vi "Send Command.vi"(8 "error in (no error)":errorcluster, 10 "Consumer Queues in":T1, 11 "Trig Process Command":refnum<class "Generic Trig Process Command.lvclass">) -> (0 "error out":errorcluster, 2 "Consumer Queues out":T1)   [LabVIEW 2019, in "Trig Process.lvlib" / "Generic Trig Process Command.lvclass"]
uses:
  Generic Trig Process Command.lvclass
  TS Framework/Consumer Queues.ctl
  UI Process/Generic UI Command/Generic UI Process Command.lvclass
  DAC Process/Generic DAC Command/Generic DAC Process Command.lvclass
  TS Framework/TS Framework.lvlib
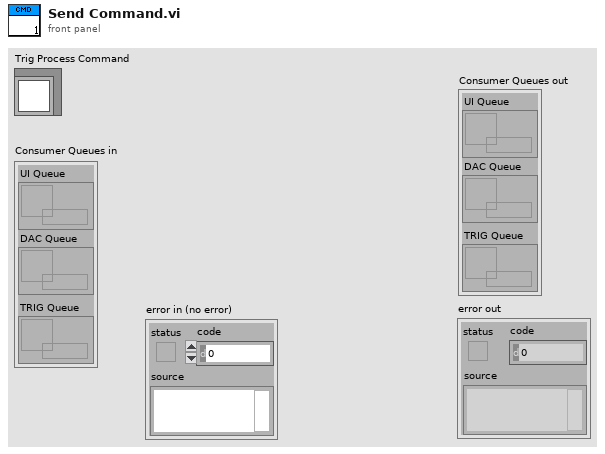
[diagram p1: front panel]
types:
  T1 = typedef "TS Framework.lvlib/Consumer Queues.ctl" = cluster{"UI Queue":refnum<queue>, "DAC Queue":refnum<queue>, "TRIG Queue":refnum<queue>}
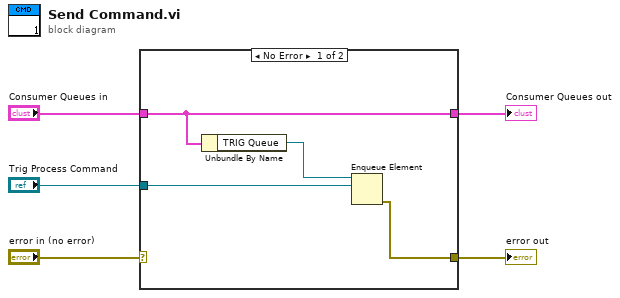
[diagram p0: block diagram]
diagram:
  n1 = case shown="No Error" "error in (no error)" {
    selector: "error in (no error)" -> [_ w11]
    tunnel: "Consumer Queues in" -> [w7 w10]
    tunnel: "Trig Process Command" -> [w8 _]
    tunnel: [w6 w11] -> w2
    tunnel: [w7 w10] -> w1
    frame No Error {
      n2 = Unbundle By Name(w7) -> ("TRIG Queue"=w9:refnum<queue>)
      n3 = Enqueue Element(queue=w9, element=w8) -> (error out=w6:errorcluster)  [unwired: 2 in, 2 out]
    }
    frame Error {
    }
  }
  "error out" <- w2
  "Consumer Queues out" <- w1
